vi "FormularFilters.vi"(6 "ImgY":i32, 7 "FilterParam":T1={"D0"=0, "D1"=0, "u0"=10, "v0"=30, "n"=1}, 8 "EorIn":errorcluster, 9 "ImgX":i32, 11 "Filter":T2(ring)) -> (0 "ErrOut":errorcluster, 1 "H(u,v)":dbl[][](array[numeric]))   [LabVIEW 2014]
doc: "Use this template to build a VI to use as a subVI."
panel:
  # "Output Parameters"
  # "Input Parameters"
  # "1) low/high pass filter controlled by D0;\n2) Band pass/reject controlled by D0(low cut) and D1(high cut);\n3) Notch Filter controlled by (+/-u0,+/-v0) and D0;"
  # "VI Description:\nThis VI is .."
  # ":: MVi Framework V1.0 ::\nAuthor:Gaoke Yang\nEmail: gaoke.yang@yahoo.com\nWeb: www.mvicontrol.com\nCopyright (C) 2015, MVI Technologies All Rights Reserved"
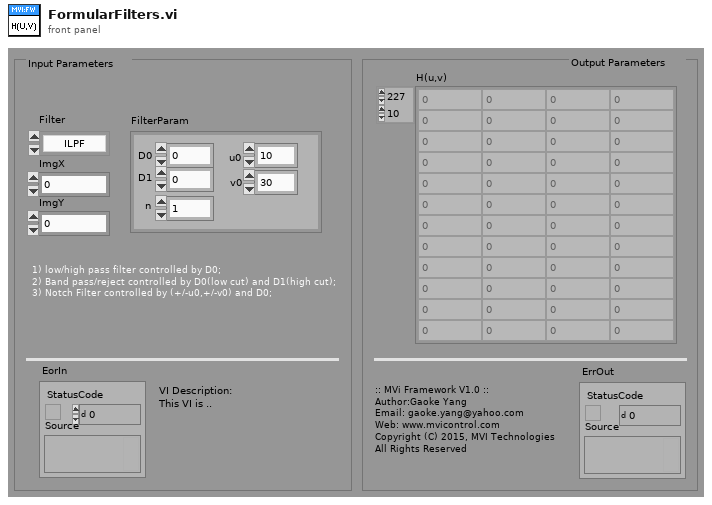
[diagram p1: front panel]
types:
  T1 = cluster{"D0":u16, "D1":u16, "u0":i16, "v0":i16, "n":u8}
  T2 = enum16{"ILPF", "IHPF", "IBPF", "IBRF", "BLPF", "BHPF", "BBPF", "BBRF", "ELPF", "EHPF", "EBPF", "EBRF", "GLPF", "GHPF", "GBPF", "GBRF"}
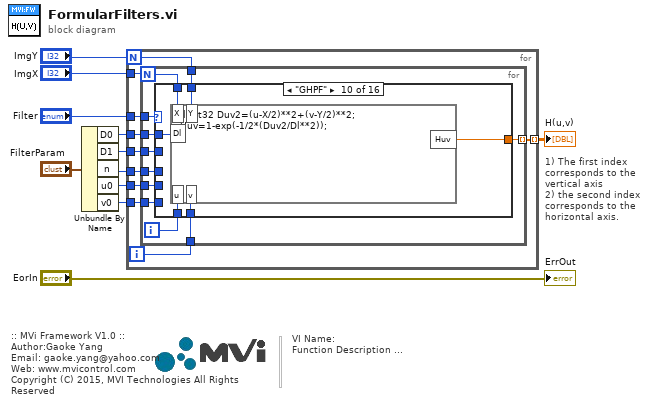
[diagram p0: block diagram]
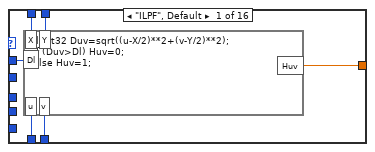
[diagram p2: hidden frame]
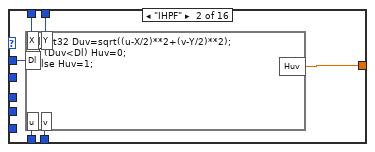
[diagram p3: hidden frame]
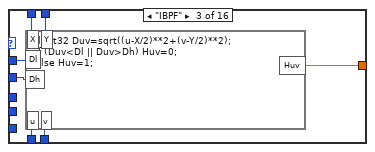
[diagram p4: hidden frame]
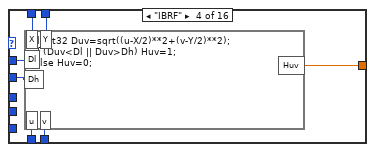
[diagram p5: hidden frame]
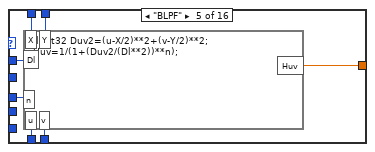
[diagram p6: hidden frame]
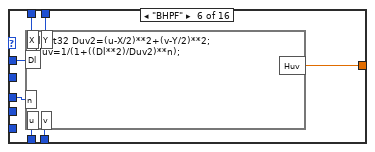
[diagram p7: hidden frame]
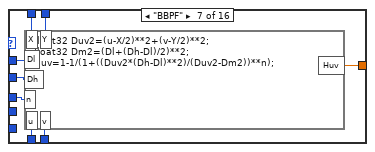
[diagram p8: hidden frame]
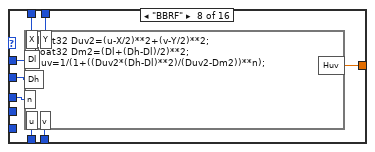
[diagram p9: hidden frame]
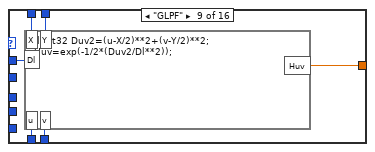
[diagram p10: hidden frame]
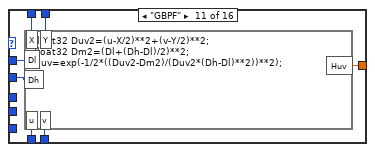
[diagram p11: hidden frame]
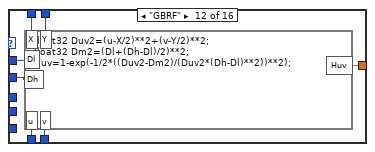
[diagram p12: hidden frame]
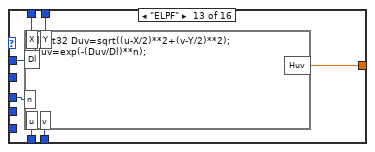
[diagram p13: hidden frame]
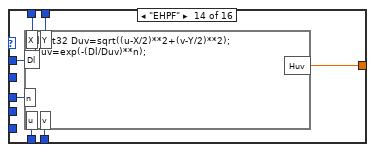
[diagram p14: hidden frame]
diagram:
  # "1) The first index corresponds to the vertical axis \n2) the second index corresponds to the horizontal axis."
  # "VI Name:\nFunction Description ..."
  # ":: MVi Framework V1.0 ::\nAuthor:Gaoke Yang\nEmail: gaoke.yang@yahoo.com\nWeb: www.mvicontrol.com\nCopyright (C) 2015, MVI Technologies All Rights Reserved"
  n1 = Unbundle By Name("FilterParam") -> ("D0"=w5:u16, "D1"=w4:u16, "n"=w3:u8, "u0"=w2:i16, "v0"=w1:i16)
  n2 = for {
    N: "ImgY" -> [w15]
    tunnel: "ImgX" -> [w21]
    tunnel: "Filter" -> [w20]
    tunnel: w5 -> [w19]
    tunnel: w4 -> [w18]
    tunnel: w3 -> [w17]
    tunnel: [w14] -> w7 mode=indexing
    tunnel: w2 -> [w13]
    tunnel: w1 -> [w12]
    i -> [w16]
    n3 = for {
      N: w21 -> [w26]
      tunnel: w20 -> [w32]
      tunnel: w19 -> [w31]
      tunnel: w18 -> [w30]
      tunnel: w17 -> [w29]
      tunnel: w16 -> [w27]
      tunnel: w15 -> [w25]
      tunnel: [w24] -> w14 mode=indexing
      tunnel: w13 -> [w23]
      tunnel: w12 -> [w22]
      i -> [w28]
      n4 = case shown="\"GHPF\"" w32 {
        tunnel: w31 -> [w35 w41 w48 w52 w65 w69 w77 w85 w89 w95 w104 w111 w116 w125 _ _]
        tunnel: w30 -> [_ _ w47 w53 _ _ w76 w84 _ _ w103 w110 _ _ _ _]
        tunnel: w29 -> [_ _ _ _ w64 w68 w75 w83 _ _ _ _ w115 w124 _ _]
        tunnel: w28 -> [w37 w42 w46 w55 w63 w67 w74 w82 w92 w98 w102 w109 w119 w123 _ _]
        tunnel: w27 -> [w36 w43 w45 w54 w62 w66 w73 w81 w91 w97 w101 w108 w118 w122 _ _]
        tunnel: w26 -> [w34 w40 w50 w57 w61 w71 w78 w86 w94 w100 w105 w112 w121 w127 _ _]
        tunnel: w25 -> [w33 w39 w49 w56 w60 w70 w79 w87 w93 w99 w106 w113 w120 w126 _ _]
        tunnel: [w38 w44 w51 w58 w59 w72 w80 w88 w90 w96 w107 w114 w117 w128 _ _] -> w24
        tunnel: w23 -> [_ _ _ _ _ _ _ _ _ _ _ _ _ _ _ _]
        tunnel: w22 -> [_ _ _ _ _ _ _ _ _ _ _ _ _ _ _ _]
        frame "ILPF", Default {
          n5 = formula code="float32 Duv=sqrt((u-X/2)**2+(v-Y/2)**2);\nif (Duv>Dl) Huv=0;\nelse Huv=1;"("u"=w37, "v"=w36, "Dl"=w35, "Y"=w33, "X"=w34) -> ("Huv"=w38:dbl)
        }
        frame "IHPF" {
          n6 = formula code="float32 Duv=sqrt((u-X/2)**2+(v-Y/2)**2);\nif (Duv<Dl) Huv=0;\nelse Huv=1;"("u"=w42, "v"=w43, "Dl"=w41, "Y"=w39, "X"=w40) -> ("Huv"=w44:dbl)
        }
        frame "IBPF" {
          n7 = formula code="float32 Duv=sqrt((u-X/2)**2+(v-Y/2)**2);\nif (Duv<Dl || Duv>Dh) Huv=0;\nelse Huv=1;"("u"=w46, "v"=w45, "Dl"=w48, "Y"=w49, "X"=w50, "Dh"=w47) -> ("Huv"=w51:dbl)
        }
        frame "IBRF" {
          n8 = formula code="float32 Duv=sqrt((u-X/2)**2+(v-Y/2)**2);\nif (Duv<Dl || Duv>Dh) Huv=1;\nelse Huv=0;"("u"=w55, "v"=w54, "Dl"=w52, "Y"=w56, "X"=w57, "Dh"=w53) -> ("Huv"=w58:dbl)
        }
        frame "BLPF" {
          n9 = formula code="float32 Duv2=(u-X/2)**2+(v-Y/2)**2;\nHuv=1/(1+(Duv2/(Dl**2))**n);"("u"=w63, "v"=w62, "Dl"=w65, "n"=w64, "Y"=w60, "X"=w61) -> ("Huv"=w59:dbl)
        }
        frame "BHPF" {
          n10 = formula code="float32 Duv2=(u-X/2)**2+(v-Y/2)**2;\nHuv=1/(1+((Dl**2)/Duv2)**n);"("u"=w67, "v"=w66, "Dl"=w69, "n"=w68, "Y"=w70, "X"=w71) -> ("Huv"=w72:dbl)
        }
        frame "BBPF" {
          n11 = formula code="float32 Duv2=(u-X/2)**2+(v-Y/2)**2;\nfloat32 Dm2=(Dl+(Dh-Dl)/2)**2;\nHuv=1-1/(1+((Duv2*(Dh-Dl)**2)/(Duv2-Dm2))**n);"("u"=w74, "v"=w73, "Dl"=w77, "n"=w75, "Y"=w79, "X"=w78, "Dh"=w76) -> ("Huv"=w80:dbl)
        }
        frame "BBRF" {
          n12 = formula code="float32 Duv2=(u-X/2)**2+(v-Y/2)**2;\nfloat32 Dm2=(Dl+(Dh-Dl)/2)**2;\nHuv=1/(1+((Duv2*(Dh-Dl)**2)/(Duv2-Dm2))**n);"("u"=w82, "v"=w81, "Dl"=w85, "n"=w83, "Y"=w87, "X"=w86, "Dh"=w84) -> ("Huv"=w88:dbl)
        }
        frame "GLPF" {
          n13 = formula code="float32 Duv2=(u-X/2)**2+(v-Y/2)**2;\nHuv=exp(-1/2*(Duv2/Dl**2));"("u"=w92, "v"=w91, "Dl"=w89, "Y"=w93, "X"=w94) -> ("Huv"=w90:dbl)
        }
        frame "GHPF" {
          n14 = formula code="float32 Duv2=(u-X/2)**2+(v-Y/2)**2;\nHuv=1-exp(-1/2*(Duv2/Dl**2));"("u"=w98, "v"=w97, "Dl"=w95, "Y"=w99, "X"=w100) -> ("Huv"=w96:dbl)
        }
        frame "GBPF" {
          n15 = formula code="float32 Duv2=(u-X/2)**2+(v-Y/2)**2;\nfloat32 Dm2=(Dl+(Dh-Dl)/2)**2;\nHuv=exp(-1/2*((Duv2-Dm2)/(Duv2*(Dh-Dl)**2))**2);"("u"=w102, "v"=w101, "Dl"=w104, "Y"=w106, "X"=w105, "Dh"=w103) -> ("Huv"=w107:dbl)
        }
        frame "GBRF" {
          n16 = formula code="float32 Duv2=(u-X/2)**2+(v-Y/2)**2;\nfloat32 Dm2=(Dl+(Dh-Dl)/2)**2;\nHuv=1-exp(-1/2*((Duv2-Dm2)/(Duv2*(Dh-Dl)**2))**2);"("u"=w109, "v"=w108, "Dl"=w111, "Y"=w113, "X"=w112, "Dh"=w110) -> ("Huv"=w114:dbl)
        }
        frame "ELPF" {
          n17 = formula code="float32 Duv=sqrt((u-X/2)**2+(v-Y/2)**2);\nHuv=exp(-(Duv/Dl)**n);"("u"=w119, "v"=w118, "Dl"=w116, "n"=w115, "Y"=w120, "X"=w121) -> ("Huv"=w117:dbl)
        }
        frame "EHPF" {
          n18 = formula code="float32 Duv=sqrt((u-X/2)**2+(v-Y/2)**2);\nHuv=exp(-(Dl/Duv)**n);"("u"=w123, "v"=w122, "Dl"=w125, "n"=w124, "Y"=w126, "X"=w127) -> ("Huv"=w128:dbl)
        }
        frame "EBPF" {
        }
        frame "EBRF" {
        }
      }
    }
  }
  "H(u,v)" <- w7
  "ErrOut" <- "EorIn"
